vi "FactoryCreate.vi"(8 "Error In":errorcluster, 10 "InstrumentConfig":T1, 11 "reference in":refnum<class "VdAnalogInput_Simulated.lvclass">) -> (0 "Error Out":errorcluster, 3 "reference out":refnum<class "VdAnalogInput_Simulated.lvclass">)   [LabVIEW 2020, in "VdAnalogInput_Simulated.lvclass"]
uses:
  VdAnalogInput_Simulated.lvclass
  VdAnalogInput_Simulated.lvclass/VdAnalogInput_Simulated.ctl
  VdInstrument_class/InstrumentType.ctl
  VdInstrument_class/VdInstrument.lvclass
  VdInstrument_class/InstrumentConfig.ctl
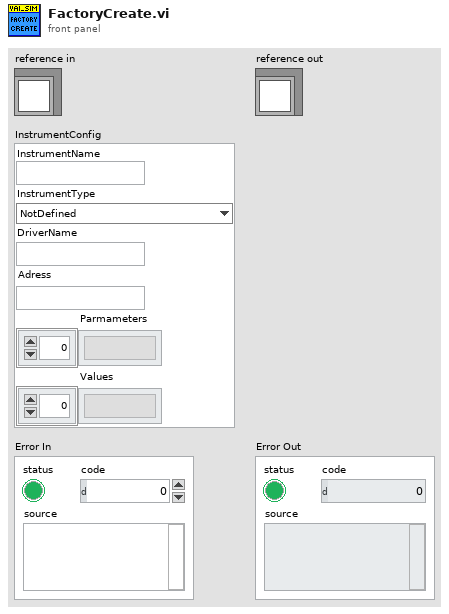
[diagram p1: front panel]
types:
  T1 = typedef "VdInstrument.lvclass/InstrumentConfig.ctl" = cluster{"InstrumentName":string, "InstrumentType":T2, "DriverName":string, "Adress":string, "Parmameters":string[], "Values":string[]}
  T2 = typedef "VdInstrument.lvclass/InstrumentType.ctl" = enum16{"NotDefined", "AirflowController", "AnalogInput", "AnalogOutput", "AutoCollimator", "BeamProfiler", "DMM", "DigitalControl", "DigitalInput", "DisplacementSensor", "Encoder", "ForceSensor", "FrequencyCounter", "FunctionGenerator", "GelDispensingRobot", "GlueDispenser", "Hexapod", "IRCamera", "ImageGenerator", "LabelPrinter", "LightController", "LightIndicator", "Load", "Multimeter", "OpticalAttenuatorPowerMeter", "OpticalChannelMonitor", "OpticalLaser", "OpticalPolarizationController", "OpticalPowerAttenuator", "OpticalPowerMeter", "OpticalSpectrumAnalyzer", "PDLMeter", "PolarisationScrambler", "PolarizationAnalyzer", "PositionSensitiveDetector", "PowerSupply", "PressureController", "Robot", "SLRCamera", "ScrewdriverController", "SignalAnalyzer", "SignalGenerator", "SixAxisStage", "SolderingStation", "SpectrumAnalyzer", "StepperMotor", "Stirrer", "SweptWavelengthSystem", "Switch", "TemperatureChamber", "TemperatureController", "TemperatureSensor", "TunableLaser", "UVCuring", "UsbHub", "VisionCamera", "WavelengthMeter", "WeldingLaser"}
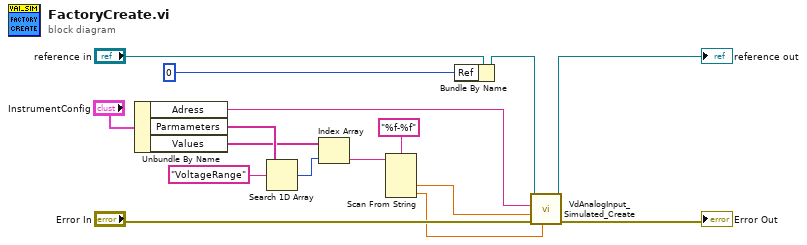
[diagram p0: block diagram]
diagram:
  n1 = Unbundle By Name("InstrumentConfig") -> ("Adress"=w9:string, "Parmameters"=w7:string[], "Values"=w6:string[])
  n2 = Search 1D Array(1D array=w7, element="VoltageRange") -> (index of element=w5:i32)  [unwired: 1 in]
  n3 = Index Array(array=w6, index=w5) -> (element=w4:string)
  n4 = Scan From String(format string="%f-%f", input string=w4) -> (output 1=w2:dbl, output 2=w1:dbl)  [unwired: 4 in, 3 out]
  n5 = Bundle By Name(cluster="reference in", "Ref"=u32 0) -> (w12:refnum<class "VdAnalogInput_Simulated.lvclass">)
  n6 = call "VdAnalogInput_Simulated_Create.vi"("VoltageRangeHigh"=w1, "Error In"="Error In", "VoltageRangeLow"=w2, "Address"=w9, "reference in"=w12) -> ("Error Out"=→"Error Out":errorcluster, "reference out"=→"reference out":refnum<class "VdAnalogInput_Simulated.lvclass">)  [unwired: 5 in]
